vi "2_Blink_Remote.vi"() -> ()   [LabVIEW 2012]
uses:
  <userlib>/BotSpeak/VIs/Scripting/URAPI_ForStart_num.vi
  <userlib>/BotSpeak/VIs/Scripting/URAPI_WriteDigitalOut_num.vi
  <userlib>/BotSpeak/VIs/Scripting/URAPI_Delay_num.vi
panel:
  out "expected response":string="start script\r\nend script\r\n................................\nDone\r\n"
  out "BotSpeak":string="SCRIPT\nSET count0,0\n\nSET DIO[1],1\nWAIT 1.000000\nSET DIO[1],0\nWAIT 1.000000\nADD count0,1\nIF (count0 < 5) GOTO 3\nend\nENDSCRIPT\nRUN&WAIT 0\n\n"
  out "response":string="start script\r\nend script\r\n................................\nDone\r\n"
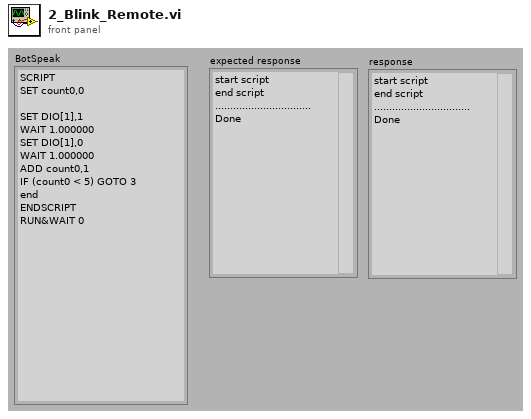
[diagram p1: front panel]
types:
  T1 = typedef "URAPI_Control.ctl" = cluster{"Script":string, "Whiles":u8[], "Ifs":u8[], "Supress Err":bool, "Errors":string}
  T2 = typedef "BotSpeak_Control.ctl" = cluster{"Address":string, "Reply EOF":string, "Hardware":path, "Retries":i8, "Timeout":i32}
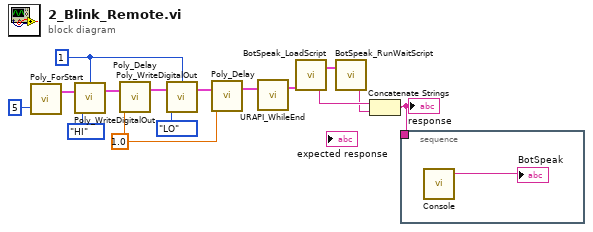
[diagram p0: block diagram]
diagram:
  w9 = sgl 1.0 ("Time In")
  w12 = u8 1 ("Channel")
  n1 = call-poly <userlib>:"Poly_ForStart.vi"("Iterations"=u16 5) -> ("URAPI Script Out"=w8:T1)  [unwired: 3 in, 1 out]
  n2 = call-poly <userlib>:"Poly_WriteDigitalOut.vi"("Value"=enum16{"LO", "HI"}."HI" ("Variable In"), "URAPI Script"=w8, "Channel"=w12) -> ("URAPI Script"=w15:T1)  [unwired: 1 in, 1 out]
  n3 = call-poly <userlib>:"Poly_Delay.vi"("Time In"=w9, "URAPI Script"=w15) -> ("URAPI Script out"=w13:T1)  [unwired: 3 in]
  n4 = call-poly <userlib>:"Poly_WriteDigitalOut.vi"("Value"=enum16{"LO", "HI"}."LO" ("Variable In"), "URAPI Script"=w13, "Channel"=w12) -> ("URAPI Script"=w14:T1)  [unwired: 1 in, 1 out]
  n5 = call-poly <userlib>:"Poly_Delay.vi"("Time In"=w9, "URAPI Script"=w14) -> ("URAPI Script out"=w7:T1)  [unwired: 3 in]
  n6 = call <userlib>:"URAPI_WhileEnd.vi"("URAPI Script"=w7) -> ("URAPI Script Out"=w5:T1)  [unwired: 4 in]
  n7 = call <userlib>:"BotSpeak_LoadScript.vi"("URAPI Script"=w5) -> ("total response"=w3:string, "Bot Settings"=w4:T2)  [unwired: 1 in]
  n8 = call <userlib>:"BotSpeak_RunWaitScript.vi"("Bot Settings"=w4) -> ("response"=w2:string)  [unwired: 1 in, 1 out]
  n9 = Concatenate Strings(w3, w2) -> (w1:string)
  "response" <- w1
  n10 = stacked-sequence {
    tunnel: w1 -> [_]
    frame #0 {
      n11 = call <userlib>:"Console.vi"() -> ("BotSpeak"=→"BotSpeak":string)  [unwired: 4 in, 1 out]
    }
  }
